vi "IFilterHome.vi"(0 "PRIORLib.IFilterIn":refnum<k7>, 1 "Filter Wheel #":i32=1) -> (2 "PRIORLib.IFilterrOut":refnum<k7>, 3 "error out":errorcluster, 4 "Return":i32)   [LabVIEW 2011]
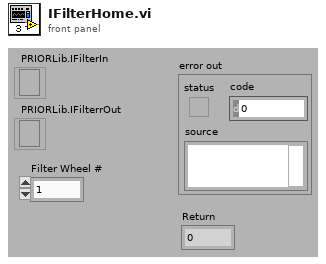
[diagram p1: front panel]
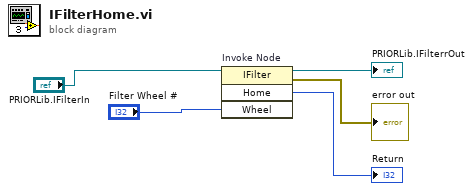
[diagram p0: block diagram]
diagram:
  n1 = invoke on="Invoke Node" class="IFilter" method="Home"(reference="PRIORLib.IFilterIn", "Wheel"="Filter Wheel #") -> (reference out=→"PRIORLib.IFilterrOut":refnum<k7>, error out=→"error out":errorcluster, "Home"=→"Return":i32)  [unwired: 2 in, 1 out]
